vi "AlliGator Get 2-Exp Guess Parameters.vi"(9 "IRF":cluster{"t Array":dbl[], "Data Array":dbl[]}, 11 "Decay":cluster{"t Array":dbl[], "Data Array":dbl[]}) -> (0 "Guess Parameters Type":T1, 1 "Guess Parameters Names":T2[](array[typedef]), 3 "Guess Parameters":dbl[](array[numeric]))   [LabVIEW 2021, in "AlliGator Decay Analysis.lvlib" / "AlliGator Decay Fit.lvlib"]
doc: "Determines <B>Guess Parameters</B> for a 2-Exp fit according to the user-specified choices:\n\n* Last valid fitted parameters:\n\nIf the number of available last valid fitted parameters is correct, uses those, otherwise use the estimated parameters.\n\n* User-provided parameters:\n\nIf a parameter is provided by the user, uses it, otherwise uses the estimated parameter.\n\n* User-provided (normalized) parameters:\n\nIf a normalized-parameter (amplitude or baseline) is provided by the user, uses it, otherwise uses the estimated parameter.\n\n* Numerically estimated parameters:\n\nUse the numerically estimated parameters."
uses:
  AlliGator Decay Fit.lvlib
  Fits/IRF(X)PSED/Decay Fit Parameters In List.ctl
  AlliGator Guess Parameters Options.ctl
  AlliGator Settings List.ctl
  Variant/Variant to Data/Variant to [DBL].vi
  <userlib>/_OpenG.lib/array/array.llb/Sort 1D Array (I16)__ogtk.vi
  <userlib>/_OpenG.lib/array/array.llb/Reorder 1D Array2 (DBL)__ogtk.vi
  AlliGator Settings.lvlib
  Variant/Variant to Data/Variant to Data.lvlib
  Fits/Fits.lvlib
  <userlib>/_OpenG.lib/array/array.llb/openg_array.lvlib
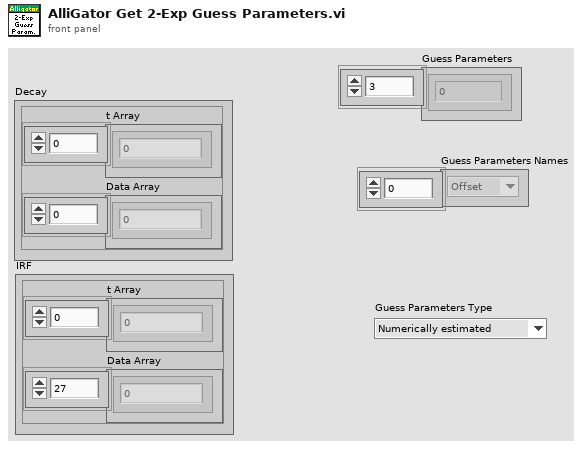
[diagram p1: front panel]
types:
  T1 = typedef "AlliGator Decay Analysis.lvlib/AlliGator Decay Fit.lvlib/AlliGator Guess Parameters Options.ctl" = enum16{"Numerically estimated", "User-provided", "User-provided (normalized)", "Last valid fitted parameters"}
  T2 = typedef "Fits.lvlib/Decay Fit Parameters In List.ctl" = enum16{"Offset", "Baseline", "A_1", "tau_1", "A_2", "tau_2"}
  T3 = typedef "AlliGator Settings.lvlib/AlliGator Settings List.ctl" = enum16{"GUI:Visible Settings Tab", "GUI:Last Run Version", "Source Image:Use Image Histogram for Contrast", "Source Image:Low Count Pixels Rejection Options", "Source Image:High Count Pixels Rejection Options", "Source Image:Use Image Brightness", "Source Image:Blend Overlay with Image Background", "Source Image:Use Fixed ROI Diameter", "Source Image:ROI Diameter", "Source Image:ROI Center Color", "Source Image:Peak Threshold", "Source Image:Intensity Threshold", "Source Image:Image Binning Options", "Source Image:Image Smoothing Options", "Source Image:Image Histogram Active", "Source Image:Invert Binary Mask", "Source Image:Hot Pixel Removal", "Source Image:Overlay Analyzed ROI Center", "Source Image:Auto-Adjust Contrast", "Source Image:Histogram Lower Percentile", "Source Image:Histogram Upper Percentile", "Source Image:Save Source Image", "Source Image:Scale Bar Options", "Source Image:Image Resolution (Pixel Size)", "Source Image:Flatfield Correction", "Source Image:Show Dead Left Columns Correction", "Source Image:Dead Left Columns Correction", "Source Image:Image Pre-Processing Operations Order", "Data Information:Gate Width", "Data Information:Nanotime Gate Separation", "Data Information:Macrotime Gate Separation", "Data Information:Gate Step", "Data Information:# Gates", "Data Information:Gate Image Exposure", "Data Information:Gate Image Integration", "Data Information:Gates to Skip", "Data Information:Gates to Keep", "Data Information:Define Gates to", "Data Information:Channel Name", "Data Information:Available Channel Names", "Data Information:Channel Arithmetic", "Data Information:Background File Subtraction", "Data Information:Background File", "Data Information:Background Scaling Factor", "Data Information:Background Pile-up Correction", "Data Information:Background Pixel Well Capacity", "Data Information:Laser Period", "Data Information:SYNC Period", "Data Information:Pile-up Correction", "Data Information:Pixel Well Capacity", "Data Information:Dataset Scaling Factor", "Fluorescence Decay_Decay Pre-Processing:Reverse Gates", "Fluorescence Decay_Decay Pre-Processing:Verbose Decay Pre-Processing", "Fluorescence Decay_Decay Pre-Processing:Use Decay Pre-Processing", "Fluorescence Decay_Decay Pre-Processing:Background Subtraction", "Fluorescence Decay_Decay Pre-Processing:Background Definition Range", "Fluorescence Decay_Decay Pre-Processing:Baseline Subtraction Method", "Fluorescence Decay_Decay Pre-Processing:Decay Pre-Processing Operations Order", "Fluorescence Decay_Decay Pre-Processing:Smoothing Parameter", "Fluorescence Decay_Decay Pre-Processing:Shift Decay", "Fluorescence Decay_Decay Pre-Processing:Decay Shift Parameters", "Fluorescence Decay_Decay Pre-Processing:Fold Decay", "Fluorescence Decay_Decay Pre-Processing:# Folds", "Fluorescence Decay_Decay Pre-Processing:1-Normalize Decay", "Fluorescence Decay_Decay Pre-Processing:[0-1]-Normalize Decay", "Fluorescence Decay_Decay Pre-Processing:Smoothen Decay", "Fluorescence Decay_Decay Pre-Processing:Extrapolate Decay", "Fluorescence Decay_Decay Pre-Processing:Use Periodicity", "Fluorescence Decay_Decay Pre-Processing:Use Cursors", "Fluorescence Decay_Decay Pre-Processing:Tail Fraction", "Fluorescence Decay_Decay Pre-Processing:Head Fraction", "Fluorescence Decay_Decay Pre-Processing:Additional Points", "Fluorescence Decay_Decay Pre-Processing:Straighten Decay", "Fluorescence Decay_Decay Pre-Processing:Constant Background", "Fluorescence Decay_Decay Pre-Processing:Pixel-Normalize Decay", "Fluorescence Decay_Advanced Analysis:Extract IRF instead of Decay", "Fluorescence Decay_Advanced Analysis:IRF Extraction Options", "Fluorescence Decay_Advanced Analysis:IRF Optimization Options", "Fluorescence Decay_Advanced Analysis:Square Pulse Options", "Fluorescence Decay_Advanced Analysis:IRF Order", "Fluorescence Decay_Advanced Analysis:IRF Time Constants", "Fluorescence Decay_Advanced Analysis:Wavelet Analysis Options", "Fluorescence Decay_Advanced Analysis:Average Lifetime Options", "Fluorescence Decay_Fit Options:Fit Options", "Fluorescence Decay_Fit Options:Use Legacy Fitting Approach", "Fluorescence Decay_Fit Options:Use Data Information Laser Period", "Fluorescence Decay_Fit Parameters:Displayed Fit Parameters", "Fluorescence Decay_Fit Parameters:Fit Parameter Constraints", "Fluorescence Decay_Fit Parameters:Export Tabulated Results", "Fluorescence Decay_Fit Parameters:MLE Baseline Offset Type", "Fluorescence Decay_Fit Parameters:MLE Baseline Offset", "Fluorescence Decay_Fit Parameters:Guess Parameter Names", "Fluorescence Decay_Fit Parameters:Guess Parameter Values", "Fluorescence Decay_Fit Parameters:Guess Parameters Options", "Fluorescence Decay_Styles:Show Last Decay Only", "Fluorescence Decay_Styles:Decay Graph Color Array", "Fluorescence Decay:Decay Graph Active", "Fluorescence Decay Statistics:Min Peak Value", "Fluorescence Decay Statistics:Reject Low Decay Peak Pixels", "Fluorescence Decay Statistics:Reject High Decay Peak Pixels", "Fluorescence Decay Statistics:Max Peak Value", "Time Traces:Use File Timestamp", "Time Traces:Time Step", "Time Traces:Use Intensity Correction File", "Time Traces:Intensity Correction File", "Phasor Plot:Phasor Plot Smoothing Options", "Phasor Plot:Phasor Plot Size", "Phasor Plot:Phasor Plot Graphics Options", "Phasor Plot:Cumulative Phasor Plot", "Phasor Plot:Use Phasor Brightness", "Phasor Plot:Blend Overlay with Phasor Background", "Phasor Plot:Save Phasor Plot", "Phasor Plot:Show References", "Phasor Plot:Phasor Ratio Decay Range", "Phasor Plot:Exponential Fading", "Phasor Plot:Phasor Ratio Reference Colors", "Phasor Plot:Reference Radius", "Phasor Plot:Show Color Map Vertices", "Phasor Plot:Phasor Plot Active", "Phasor Plot:Phasor Ratio Color Map Type", "Phasor Plot:Phasor Ratio Color Map", "Phasor Plot:Phasor Ratio Display Range", "Phasor Plot:Selected Image ROI(s)", "Phasor Plot:All Image ROIs", "Phasor Plot:Selected Phasor Plot ROI(s)", "Phasor Plot:All Phasor Plot ROIs", "Phasor Plot:Phasor Ratio Color-Coded Quantity", "Phasor Plot:Store Phasor Harmonics", "Phasor Plot:Draw Reference Segment", "Phasor Plot:User-Defined Quantity", "Phasor Graph:Phasor Frequency", "Phasor Graph:Phasor Ratio Type", "Phasor Graph:Pixel-level Phasor Computation", "Phasor Graph:Save Phasor Graph", "Phasor Graph:Phasor Graph Active", "Phasor Graph:Phasor SDV Options", "Phasor Calibration:Use Backup Calibration if needed", "Phasor Graph:Define Shortest Lifetime as", "Phasor Calibration:Backup Calibration Type", "Phasor Calibration:Calibration Type", "Phasor Calibration:Calibration Lifetime", "Phasor Calibration:Calibration Map Algorithm", "Single-Exponential Phasor Locus (SEPL):Gate Parameters", "Single-Exponential Phasor Locus (SEPL):User-defined Gate", "Single-Exponential Phasor Locus (SEPL):User-defined IRF", "Single-Exponential Phasor Locus (SEPL):Phasor Parameters", "Single-Exponential Phasor Locus (SEPL):Decay & IRF Parameters", "Single-Exponential Phasor Locus (SEPL):Display Parameters", "Lifetime Analysis:Decay Analysis Parameters", "Lifetime Analysis:Lifetime Map Active", "Plugins:Python Settings", "Miscellaneous:Verbose Mode", "Miscellaneous:Beep after Script", "Miscellaneous:Saved Image File Format", "Miscellaneous:Exported Gate Image Settings", "Miscellaneous:Include Loading in Timing", "Miscellaneous:Verbose Settings Mode", "Miscellaneous:Histogram Options", "Miscellaneous:Beep on Error", "Miscellaneous:# Logical Processors Used", "Miscellaneous:ROI Description Max Characters", "Miscellaneous:Verbose Error Mode", "Miscellaneous:Transparent Mask Color"}
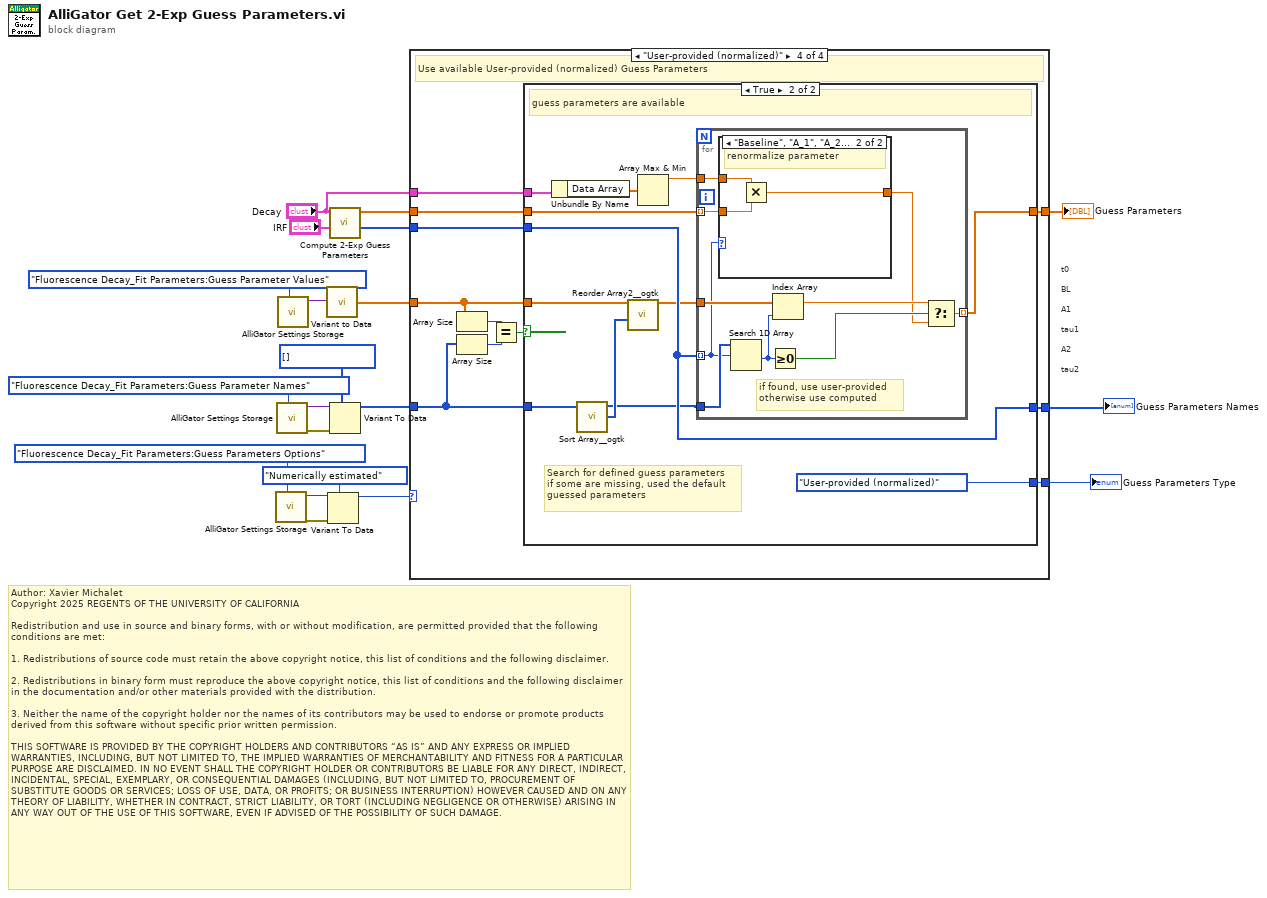
[diagram p0: block diagram]
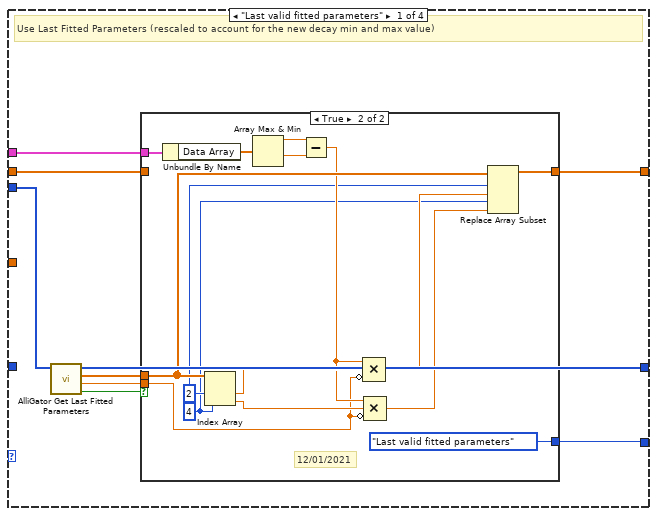
[diagram p2: hidden frame]
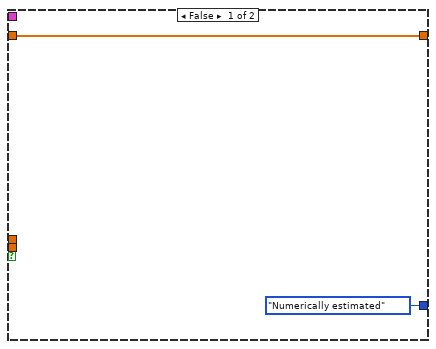
[diagram p3: hidden frame]
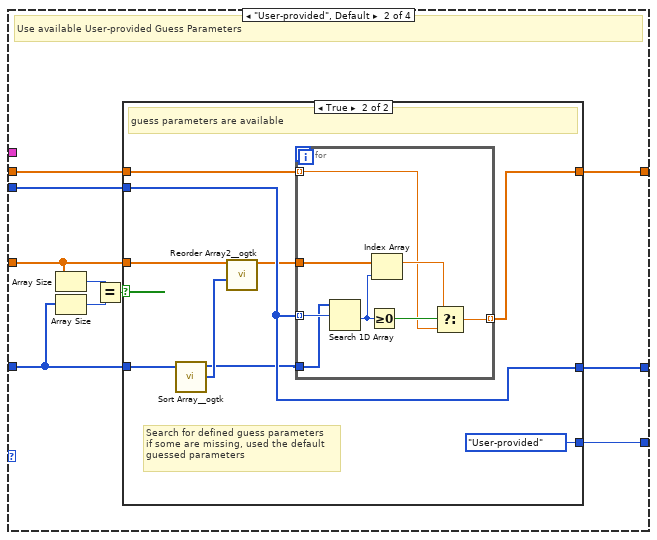
[diagram p4: hidden frame]
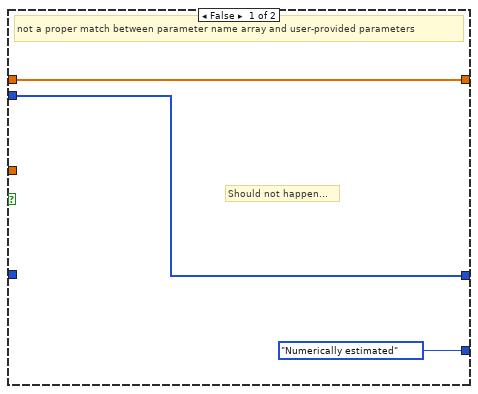
[diagram p5: hidden frame]
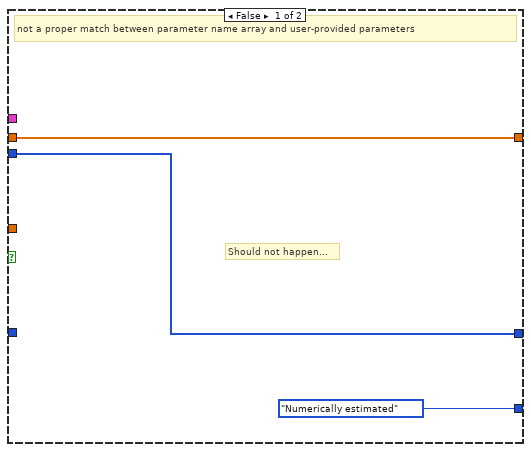
[diagram p7: hidden frame]
diagram:
  w15 = T2[] [] items=["Offset", "Baseline", "A_1", "tau_1", "A_2", "tau_2"] ("Guess Parameters Names")
  # "Author: Xavier Michalet\nCopyright 2025 REGENTS OF THE UNIVERSITY OF CALIFORNIA\n\nRedistribution and use in source and binary forms, with or without modification, are permitted provided that the following conditions are met:\n\n1. Redistributions of source code must retain the above copyright notice, this list of conditions and the following disclaimer.\n\n2. Redistributions in binary form must reproduce the above copyright notice, this list of conditions and the following disclaimer in the documentation and/or other materials provided with the distribution.\n\n3. Neither the name of the copyright holder nor the names of its contributors may be used to endorse or promote products derived from this software without specific prior written permission.\n\nTHIS SOFTWARE IS PROVIDED BY THE COPYRIGHT HOLDERS AND CONTRIBUTORS “AS IS” AND ANY EXPRESS OR IMPLIED WARRANTIES, INCLUDING, BUT NOT LIMITED TO, THE IMPLIED WARRANTIES OF MERCHANTABILITY AND FITNESS FOR A PARTICULAR PURPOSE ARE DISCLAIMED. IN NO EVENT SHALL THE COPYRIGHT HOLDER OR CONTRIBUTORS BE LIABLE FOR ANY DIRECT, INDIRECT, INCIDENTAL, SPECIAL, EXEMPLARY, OR CONSEQUENTIAL DAMAGES (INCLUDING, BUT NOT LIMITED TO, PROCUREMENT OF SUBSTITUTE GOODS OR SERVICES; LOSS OF USE, DATA, OR PROFITS; OR BUSINESS INTERRUPTION) HOWEVER CAUSED AND ON ANY THEORY OF LIABILITY, WHETHER IN CONTRACT, STRICT LIABILITY, OR TORT (INCLUDING NEGLIGENCE OR OTHERWISE) ARISING IN ANY WAY OUT OF THE USE OF THIS SOFTWARE, EVEN IF ADVISED OF THE POSSIBILITY OF SUCH DAMAGE."
  # "t0\n\nBL\n\nA1\n\ntau1\n\nA2\n\ntau2"
  n1 = call "AlliGator Settings Storage.vi"("AlliGator Settings List"=AlliGator_Settings_List."Fluorescence Decay_Fit Parameters:Guess Parameters Options") -> ("Error Out"=w4:errorcluster, "Variant Data out"=w5:variant)  [unwired: 9 in]
  n2 = call "AlliGator Settings Storage.vi"("AlliGator Settings List"=AlliGator_Settings_List."Fluorescence Decay_Fit Parameters:Guess Parameter Names") -> ("Error Out"=w16:errorcluster, "Variant Data out"=w17:variant)  [unwired: 9 in]
  n3 = call "AlliGator Settings Storage.vi"("AlliGator Settings List"=AlliGator_Settings_List."Fluorescence Decay_Fit Parameters:Guess Parameter Values") -> ("Variant Data out"=w20:variant)  [unwired: 9 in, 1 out]
  n4 = call-poly "Variant to Data.vi"("Variant"=w20) -> ("Value"=w13:dbl[])  [unwired: 8 in]
  n5 = Variant To Data(error in=w4, type=AlliGator_Guess_Parameters_Options."Numerically estimated" ("Guess Parameters Options"), Variant=w5) -> (data=w2:T1)  [unwired: 1 out]
  n6 = call "Compute 2-Exp Guess Parameters.vi"("IRF"="IRF", "Decay"="Decay") -> ("Ordered Guess Parameter Names"=w10:T2[], "Guess Parameters"=w12:dbl[])  [unwired: 8 in]
  n7 = Variant To Data(error in=w16, type=w15, Variant=w17) -> (data=w14:T2[])  [unwired: 1 out]
  n8 = case shown="\"User-provided (normalized)\"" w2 {
    selector: w2 -> [_ _ w77 _]
    tunnel: w14 -> [_ w53 _ w87]
    tunnel: w13 -> [_ w52 _ w86]
    tunnel: w12 -> [w26 w51 w79 w85]
    tunnel: [w27 w50 w79 w84] -> w11
    tunnel: w10 -> [w24 w49 w78 w83]
    tunnel: [w25 w48 w78 w82] -> w9
    tunnel: "Decay" -> [w23 _ _ w80]
    tunnel: [w21 w47 w77 w81] -> w1
    frame "Last valid fitted parameters" {
      # "Use Last Fitted Parameters (rescaled to account for the new decay min and max value)"
      n9 = call "AlliGator Get Last Fitted Parameters.vi"("Guess Parameters Names"=w24) -> ("Last Fitted Parameters OK"=w28:bool, "Last Decay Max - Min"=w22:dbl, "Last Fitted Parameters"=w29:dbl[], "Guess Parameters Names (dup)"=w25:T2[])  [unwired: 7 in]
      n10 = case shown="True" w28 {
        tunnel: w29 -> [_ w41]
        tunnel: [w31 w43] -> w27
        tunnel: w26 -> [w31 _]
        tunnel: w23 -> [_ w44]
        tunnel: w22 -> [_ w33]
        tunnel: [AlliGator_Guess_Parameters_Options."Numerically estimated" ("Guess Parameters Type") AlliGator_Guess_Parameters_Options."Last valid fitted parameters" ("Guess Parameters Type")] -> w21
        frame False {
        }
        frame True {
          w34 = 4 ("index")
          w35 = 2 ("index")
          # "12/01/2021"
          n11 = Unbundle By Name(w44) -> ("Data Array"=w46:dbl[])
          n12 = Index Array(array=w41, index #1=w35, index #2=w34) -> (element #1=w40:dbl, element #2=w39:dbl)
          n13 = Array Max & Min(array=w46) -> (max value=w45:dbl, min value=w42:dbl)  [unwired: 2 out]
          n14 = Subtract(x=w45, y=w42) -> (x-y=w38:dbl)
          n15 = Compound Arithmetic op=MULTIPLY(w38, w40, invert w33) -> (w37:dbl)
          n16 = Compound Arithmetic op=MULTIPLY(w38, w39, invert w33) -> (w36:dbl)
          n17 = Replace Array Subset(array=w41, new element #1=w37, index #1=w35, new element #2=w36, index #2=w34) -> (w43:dbl[])
        }
      }
    }
    frame "User-provided", Default {
      # "Use available User-provided Guess Parameters"
      n18 = Array Size(array=w52) -> (size(s)=w54:i32)
      n19 = Array Size(array=w53) -> (size(s)=w56:i32)
      n20 = Equal?(x=w54, y=w56) -> (x = y?=w55:bool)
      n21 = case shown="True" w55 {
        tunnel: w53 -> [_ w64]
        tunnel: w52 -> [_ w62]
        tunnel: w51 -> [w59 w67]
        tunnel: [w59 w68] -> w50
        tunnel: w49 -> [w58 w66]
        tunnel: [w58 w66] -> w48
        tunnel: [AlliGator_Guess_Parameters_Options."Numerically estimated" ("Guess Parameters Type") AlliGator_Guess_Parameters_Options."User-provided" ("Guess Parameters Type")] -> w47
        frame False {
          # "Should not happen..."
          # "not a proper match between parameter name array and user-provided parameters"
        }
        frame True {
          # "Search for defined guess parameters\nif some are missing, used the default\nguessed parameters"
          # "guess parameters are available"
          n22 = call-poly <userlib>:"Sort Array__ogtk.vi"("Array in"=w64) -> ("Sorted Pointers"=w65:i32[], "Sorted Array out"=w63:i16[])  [unwired: 9 in]
          n23 = call-poly <userlib>:"Reorder Array2__ogtk.vi"("indices"=w65, "array"=w62) -> ("reordered array"=w61:dbl[])  [unwired: 9 in]
          n24 = for {
            tunnel: w61 -> [w73]
            tunnel: w63 -> [w75]
            tunnel: w66 -> [w76] mode=indexing
            tunnel: [w70] -> w68 mode=indexing
            tunnel: w67 -> [w69] mode=indexing
            n25 = Search 1D Array(1D array=w75, element=w76) -> (index of element=w71:i32)  [unwired: 1 in]
            n26 = Greater Or Equal To 0?(x=w71) -> (x >= 0?=w74:bool)
            n27 = Index Array(array=w73, index=w71) -> (element=w72:dbl)
            n28 = Select(t=w72, s=w74, f=w69) -> (s? t:f=w70:dbl)
          }
        }
      }
    }
    frame "Numerically estimated" {
      # "Numerically estimated"
    }
    frame "User-provided (normalized)" {
      # "Use available User-provided (normalized) Guess Parameters"
      n29 = Array Size(array=w86) -> (size(s)=w88:i32)
      n30 = Array Size(array=w87) -> (size(s)=w90:i32)
      n31 = Equal?(x=w88, y=w90) -> (x = y?=w89:bool)
      n32 = case shown="True" w89 {
        tunnel: w87 -> [_ w101]
        tunnel: w86 -> [_ w99]
        tunnel: w85 -> [w93 w104]
        tunnel: [w93 w105] -> w84
        tunnel: w83 -> [w92 w103]
        tunnel: [w92 w103] -> w82
        tunnel: [AlliGator_Guess_Parameters_Options."Numerically estimated" ("Guess Parameters Type") AlliGator_Guess_Parameters_Options."User-provided (normalized)" ("Guess Parameters Type")] -> w81
        tunnel: w80 -> [_ w96]
        frame False {
          # "Should not happen..."
          # "not a proper match between parameter name array and user-provided parameters"
        }
        frame True {
          # "Search for defined guess parameters\nif some are missing, used the default\nguessed parameters"
          # "guess parameters are available"
          n33 = Unbundle By Name(w96) -> ("Data Array"=w95:dbl[])
          n34 = call-poly <userlib>:"Sort Array__ogtk.vi"("Array in"=w101) -> ("Sorted Pointers"=w102:i32[], "Sorted Array out"=w100:i16[])  [unwired: 9 in]
          n35 = call-poly <userlib>:"Reorder Array2__ogtk.vi"("indices"=w102, "array"=w99) -> ("reordered array"=w98:dbl[])  [unwired: 9 in]
          n36 = Array Max & Min(array=w95) -> (max value=w94:dbl)  [unwired: 3 out]
          n37 = for {
            tunnel: w98 -> [w113]
            tunnel: w100 -> [w115]
            tunnel: w103 -> [w106] mode=indexing
            tunnel: [w110] -> w105 mode=indexing
            tunnel: w104 -> [w108] mode=indexing
            tunnel: w94 -> [w109]
            # "if found, use user-provided\notherwise use computed"
            n38 = case shown="\"Baseline\", \"A_1\", \"A_2\"" w106 {
              tunnel: w109 -> [_ w119]
              tunnel: w108 -> [w116 w118]
              tunnel: [w116 w117] -> w107
              frame "Offset", Default {
              }
              frame "Baseline", "A_1", "A_2" {
                # "renormalize parameter"
                n39 = Multiply(x=w119, y=w118) -> (x*y=w117:dbl)
              }
            }
            n40 = Search 1D Array(1D array=w115, element=w106) -> (index of element=w111:i32)  [unwired: 1 in]
            n41 = Greater Or Equal To 0?(x=w111) -> (x >= 0?=w114:bool)
            n42 = Index Array(array=w113, index=w111) -> (element=w112:dbl)
            n43 = Select(t=w112, s=w114, f=w107) -> (s? t:f=w110:dbl)
          }
        }
      }
    }
  }
  "Guess Parameters" <- w11
  "Guess Parameters Names" <- w9
  "Guess Parameters Type" <- w1
